vi "ZCR - array.vi"(10 "Range":i32, 11 "Input":dbl[](array[numeric])) -> (3 "Output":dbl[](array[numeric]))   [LabVIEW 2020, in "Library Commun.lvlib" / "Nodon_ZCR.lvclass"]
uses:
  Nodon_ZCR.lvclass
  Nodon_ZCR.lvclass/Nodon_ZCR.ctl
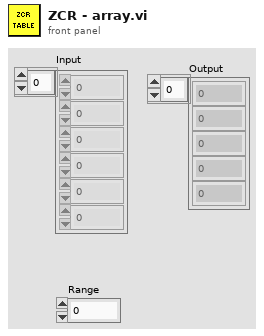
[diagram p1: front panel]
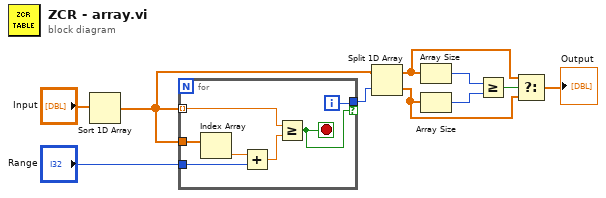
[diagram p0: block diagram]
diagram:
  n1 = Sort 1D Array(array="Input") -> (sorted array=w8:dbl[])
  n2 = for {
    tunnel: w8 -> [w13] mode=indexing
    tunnel: w8 -> [w17]
    tunnel: "Range" -> [w15]
    tunnel: [w12] -> w7 if=w11
    i -> [w12]
    stop <- w11 stop-if-true
    n3 = Index Array(array=w17) -> (element=w16:dbl)  [unwired: 1 in]
    n4 = Add(x=w16, y=w15) -> (x+y=w14:dbl)
    n5 = Greater Or Equal?(x=w13, y=w14) -> (x >= y?=w11:bool)
  }
  n6 = Split 1D Array(array=w8, index=w7) -> (first subarray=w2:dbl[], second subarray=w3:dbl[])
  n7 = Array Size(array=w2) -> (size(s)=w6:i32)
  n8 = Array Size(array=w3) -> (size(s)=w5:i32)
  n9 = Greater Or Equal?(x=w6, y=w5) -> (x >= y?=w4:bool)
  n10 = Select(t=w2, s=w4, f=w3) -> (s? t:f=→"Output":dbl[])
